vi "insert_single.vi"(7 "connection_reference":T1, 8 "error in (no error)":errorcluster, 10 "value":dbl, 11 "date_time":dbl format="%<%H:%M:%S%3u %m/%d/%y>T") -> (0 "error out":errorcluster)   [LabVIEW 2015, in "lv-example-postgres.lvlib"]
uses:
  lv-example-postgres.lvlib
  <vilib>/addons/database/Connection.llb/Conn ObjectReference.ctl
  <vilib>/addons/database/Command.llb/Cmd Execute.vi
  <vilib>/addons/database/Recordset.llb/Rec Destroy - Command.vi
  <vilib>/addons/database/Command.llb/Cmd Delete.vi
  <vilib>/addons/database/NI_Database_API.lvlib
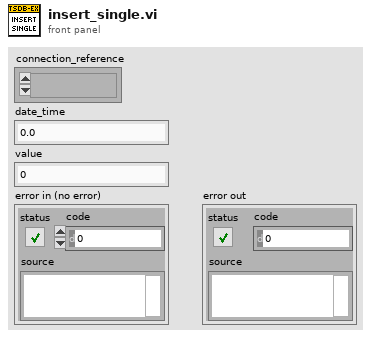
[diagram p1: front panel]
types:
  T1 = typedef "NI_Database_API.lvlib/Conn ObjectReference.ctl" = refnum<k1>
  T2 = typedef "NI_Database_API.lvlib/DB Tools Parameter Info.ctl" = cluster{"parameter name":string, "type":T3, "direction":T4, "value":variant}
  T3 = typedef "NI_Database_API.lvlib/DB Tools DataTypes.ctl" = enum16{"String", "Long (I32)", "Single (SGL)", "Double (DBL)", "Date/Time", "Binary"}
  T4 = typedef "NI_Database_API.lvlib/DB Tools Parameter Dir.ctl" = enum32{"Input", "Output", "Input/Output", "Return Value"}
  T5 = typedef "NI_Database_API.lvlib/Cmd ObjectReference.ctl" = refnum<k1>
  T6 = typedef "NI_Database_API.lvlib/Cmd-Rec Object Reference.ctl" = refnum<k1>
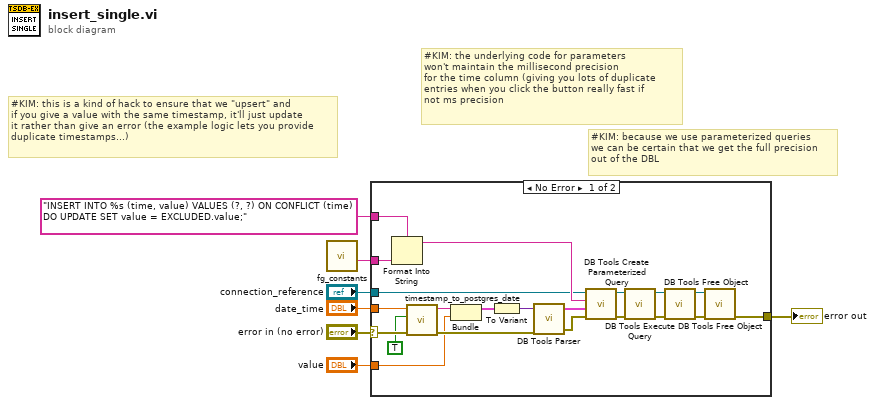
[diagram p0: block diagram]
diagram:
  # "#KIM: this is a kind of hack to ensure that we \"upsert\" and\nif you give a value with the same timestamp, it'll just update\nit rather than give an error (the example logic lets you provide\nduplicate timestamps...)"
  # "#KIM: because we use parameterized queries\nwe can be certain that we get the full precision\nout of the DBL"
  # "#KIM: the underlying code for parameters\nwon't maintain the millisecond precision\nfor the time column (giving you lots of duplicate\nentries when you click the button really fast if\nnot ms precision"
  n1 = call "fg_constants.vi"() -> ("table out"=w1:string)  [unwired: 9 in, 2 out]
  n2 = case shown="No Error" "error in (no error)" {
    selector: "error in (no error)" -> [w27 w29]
    tunnel: "INSERT INTO %s (time, value) VALUES (?, ?) ON CONFLICT (time) DO UPDATE SET value = EXCLUDED.value;" ("format string") -> [w26 _]
    tunnel: "value" -> [w25 _]
    tunnel: "date_time" -> [w24 _]
    tunnel: w1 -> [w21 _]
    tunnel: "connection_reference" -> [w14 _]
    tunnel: [w13 w29] -> w3
    frame No Error {
      n3 = Format Into String(format string=w26, w21) -> (resulting string=w20:string)  [unwired: 2 in, 1 out]
      n4 = call "timestamp_to_postgres_date.vi"("error in (no error)"=w27, "utc"=TRUE, "date_time"=w24) -> ("error out"=w28:errorcluster, "postgres_date"=w23:string)  [unwired: 7 in]
      n5 = Bundle("postgres_date"=w23, "value"=w25) -> (w19:cluster{"postgres_date":string, "value":dbl})  [unwired: 1 in]
      n6 = To Variant(anything=w19) -> (Variant=w8:variant)
      n7 = call <vilib>:"DB Tools Parser.vi"("error in (no error)"=w28, "variant"=w8) -> ("error out"=w18:errorcluster, "parameters"=w9:T2[])  [unwired: 2 in]
      n8 = call <vilib>:"DB Tools Create Parameterized Query.vi"("error in (no error)"=w18, "parameters"=w9, "SQL query"=w20, "connection reference"=w14) -> ("error out"=w11:errorcluster, "command reference"=w15:T5)  [unwired: 3 in, 1 out]
      n9 = call-poly <vilib>:"DB Tools Execute Query.vi"("error in (no error)"=w11, "command reference"=w15) -> ("error out"=w10:errorcluster, "command-recordset reference"=w16:T6)  [unwired: 6 in]
      n10 = call-poly <vilib>:"DB Tools Free Object.vi"("error in (no error)"=w10, "command-recordset reference"=w16) -> ("error out"=w12:errorcluster, "command reference"=w17:T5)  [unwired: 8 in]
      n11 = call-poly <vilib>:"DB Tools Free Object.vi"("error in (no error)"=w12, "command reference"=w17) -> ("error out"=w13:errorcluster)  [unwired: 8 in, 1 out]
    }
    frame Error {
    }
  }
  "error out" <- w3
